vi "Set Item by name.vi"(8 "error in (no error)":errorcluster, 9 "Value":refnum<class "JSON Value.lvclass">, 10 "name":string, 11 "JSON Object in":refnum<class "JSON Object.lvclass">) -> (0 "error out":errorcluster, 2 "replaced":bool, 3 "JSON Object out":refnum<class "JSON Object.lvclass">)   [LabVIEW 2011, in "JSON Object.lvclass"]
doc: "Stores a <b>JSON Value</b> in a <b>JSON Object</b> by it's name.\n\nCopyright 2012 James David Powell, Shaun Rumbell and Ton Plomp\nMore information on http://lavag.org/topic/16217-cr-json-labview"
uses:
  JSON Object.lvclass
  JSON Value/JSON Value.lvclass
  JSON Object.lvclass/JSON Object.ctl
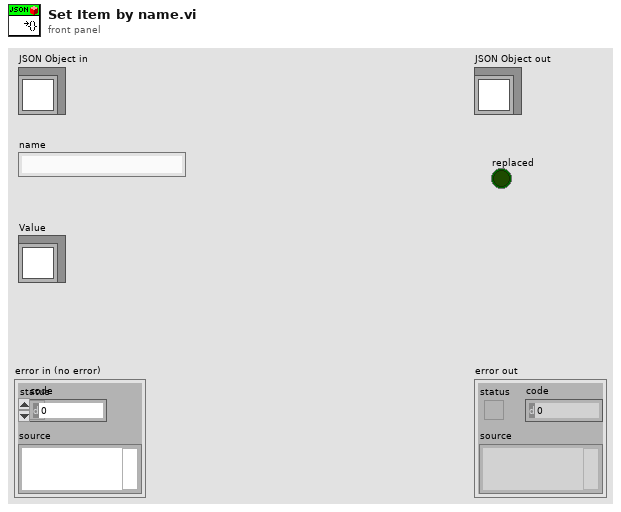
[diagram p1: front panel]
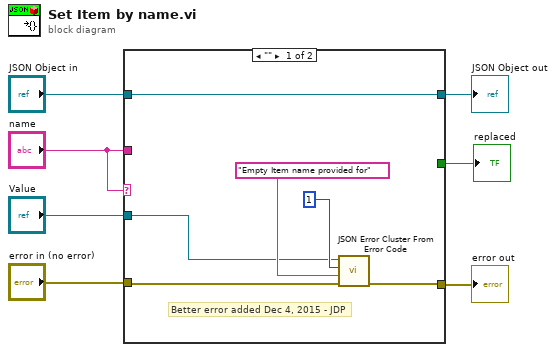
[diagram p0: block diagram]
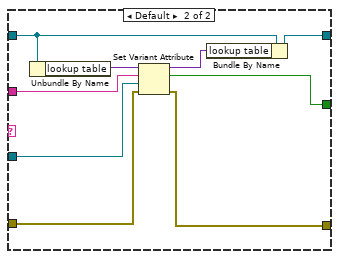
[diagram p2: hidden frame]
diagram:
  n1 = case shown="\"\"" "name" {
    tunnel: "JSON Object in" -> [w13 w22]
    tunnel: "name" -> [_ w20]
    tunnel: "Value" -> [w8 w19]
    tunnel: "error in (no error)" -> [w9 w18]
    tunnel: [w10 w17] -> w4
    tunnel: [_ w16] -> w3
    tunnel: [w13 w15] -> w2
    frame "" {
      # "Better error added Dec 4, 2015 - JDP"
      n2 = call "JSON Error Cluster From Error Code.vi"("error in (no error)"=w9, "Error message"="Empty Item name provided for", "JSON error code"=1, "JSON Value in"=w8) -> ("error out"=w10:errorcluster)  [unwired: 6 in, 1 out]
    }
    frame Default {
      n3 = Unbundle By Name(w22) -> ("lookup table"=w21:variant)
      n4 = Set Variant Attribute(Variant=w21, name=w20, value=w19, error in=w18) -> (Variant out=w14:variant, replaced=w16:bool, error out=w17:errorcluster)
      n5 = Bundle By Name(cluster=w22, "lookup table"=w14) -> (w15:refnum<class "JSON Object.lvclass">)
    }
  }
  "error out" <- w4
  "JSON Object out" <- w2
  "replaced" <- w3
